vi "initiate.vi"(0 "reference in":refnum<class "File Controller.lvclass">, 5 "error in (no error)":errorcluster) -> (14 "reference out":refnum<class "File Controller.lvclass">, 19 "error out":errorcluster)   [LabVIEW 2015, in "File Controller.lvclass"]
uses:
  File Controller.lvclass
  APP/python_class/python.lvclass
  APP/excelFile_class/excelFile.lvclass
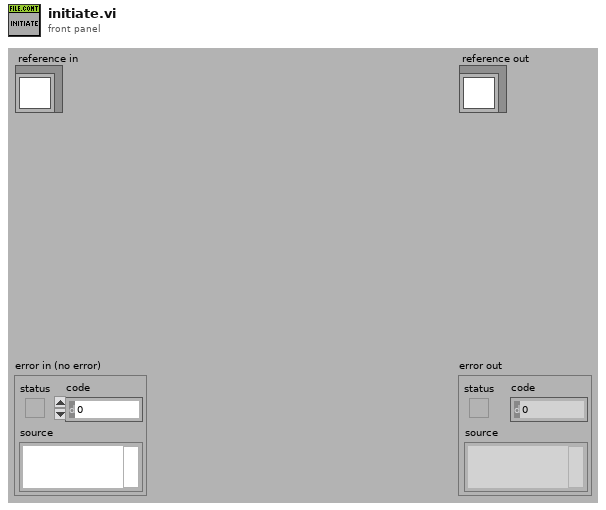
[diagram p1: front panel]
types:
  T1 = typedef "File Controller.lvclass/ObjectAttributesRef.ctl" = refnum<data-value>
  T2 = typedef "File Controller.lvclass/ObjectAttributes.ctl" = cluster{"MyAttribute":dbl, "excelFile_refs":refnum<class "excelFile.lvclass">[], "filePaths":path[], "outlookTemplatePaths":path[], "attachmentTemplatePaths":path[], "configFilePath":path, "not_setting":bool[], "python_ref":refnum<class "python.lvclass">}
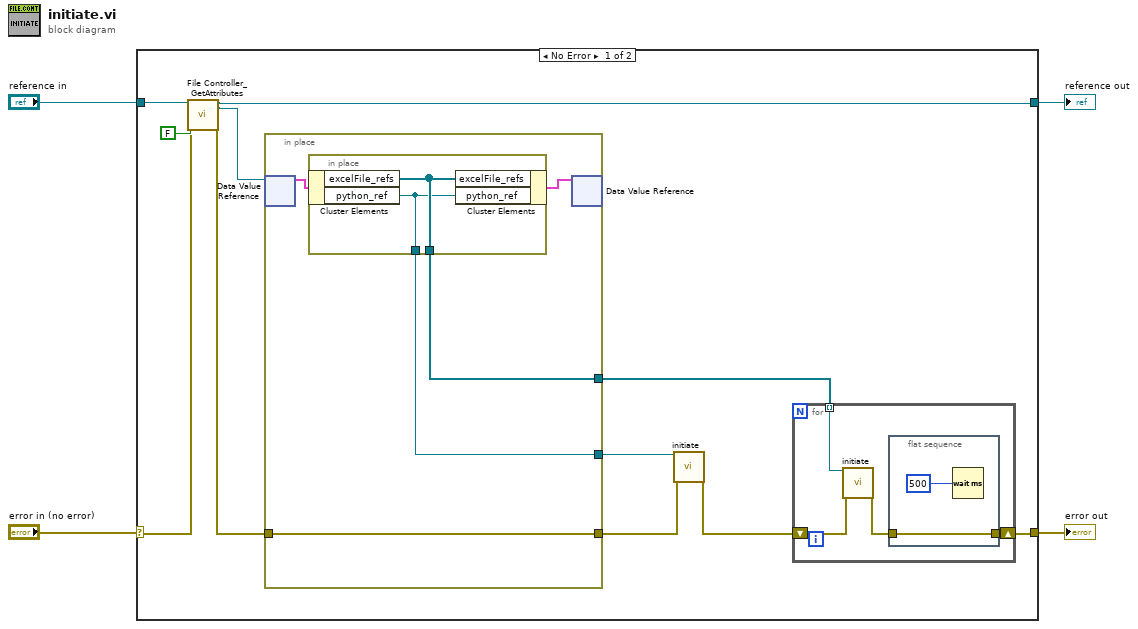
[diagram p0: block diagram]
diagram:
  n1 = case shown="No Error" "error in (no error)" {
    selector: "error in (no error)" -> [w14 w30]
    tunnel: [w8 w30] -> w3
    tunnel: [w12 w29] -> w1
    tunnel: "reference in" -> [w13 w29]
    frame No Error {
      n2 = call "File Controller_GetAttributes.vi"("reference in"=w13, "return data? (T)"=FALSE, "error in (no error)"=w14) -> ("reference out"=w12:refnum<class "File Controller.lvclass">, "attributes ref"=w10:T1, "error out"=w11:errorcluster)  [unwired: 13 in, 1 out]
      n3 = in-place {
        in-place-border: w11 -> [w24]
        in-place-border: [w24] -> w6
        in-place-border: [w23] -> w9
        in-place-border: [w22] -> w7
        n4 = in-place-dvr #1(w10) -> (w25:T2)  [unwired: 1 out]
        n5 = in-place {
          in-place-border: [w28] -> w23
          in-place-border: [w27] -> w22
          n6 = in-place-cluster #2(w25) -> ("excelFile_refs"=w28:refnum<class "excelFile.lvclass">[], "python_ref"=w27:refnum<class "python.lvclass">)
          n7 = in-place-cluster #2("excelFile_refs"=w28, "python_ref"=w27) -> (w26:T2)
        }
        n8 = in-place-dvr #1(w26) -> ()  [unwired: 2 out]
      }
      n9 = call-dynamic "initiate.vi"("reference in"=w7, "error in (no error)"=w6) -> ("error out"=w5:errorcluster)  [unwired: 16 in, 1 out]
      n10 = for {
        tunnel: w9 -> [w19] mode=indexing
        shift-right: [w16] -> w8
        shift-left: w5 -> [w18]
        n11 = call-dynamic "initiate.vi"("reference in"=w19, "error in (no error)"=w18) -> ("error out"=w17:errorcluster)  [unwired: 16 in, 1 out]
        n12 = flat-sequence {
          tunnel: w17 -> [w21]
          tunnel: [w21] -> w16
          frame #0 {
            n13 = Wait (ms)(milliseconds to wait=u32 500) -> ()  [unwired: 1 out]
          }
        }
      }
    }
    frame Error {
    }
  }
  "error out" <- w3
  "reference out" <- w1
